vi "Init Search Page.vi"(7 "Next Button":refnum<vi>, 9 "\"Tab Backward To\" Refnum":refnum<vi>, 10 "\"Tab Forward To\" Refnum":refnum<vi>, 11 "SubPanel":refnum<vi>) -> (0 "Additional Search Ref":refnum<vi>, 1 "Next! Ref":refnum<vi>, 2 "Starter App Ref":refnum<vi>, 3 "Search Page Ref":refnum<vi>, 4 "SearchPage Ctrl #n Ref":refnum<vi>, 6 "SearchPage Ctrl #1 Ref":refnum<vi>)   [LabVIEW 2016]
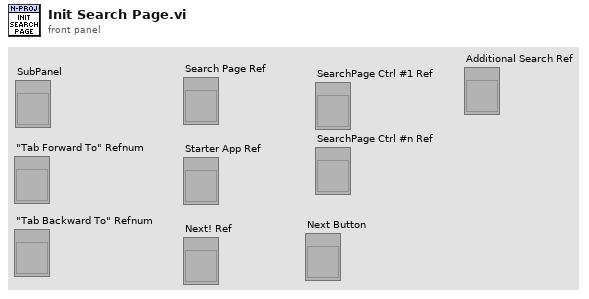
[diagram p1: front panel]
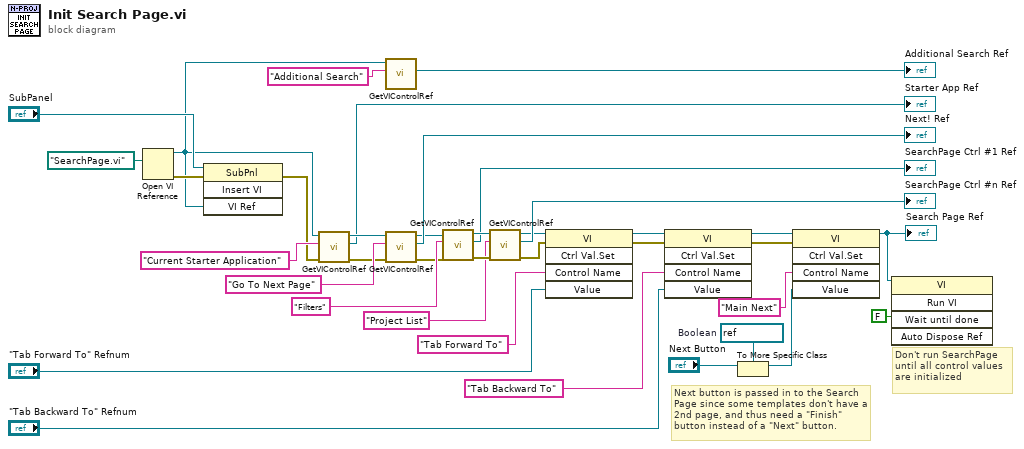
[diagram p0: block diagram]
diagram:
  w1 = refnum<vi> refnum  # Boolean
  # "Don't run SearchPage\nuntil all control values\nare initialized"
  # "Next button is passed in to the Search Page since some templates don't have a 2nd page, and thus need a \"Finish\" button instead of a \"Next\" button."
  n1 = Open VI Reference(vi path=path "SearchPage.vi") -> (vi reference=w7:refnum<vi>, error out=w29:errorcluster)  [unwired: 5 in]
  n2 = invoke on="Invoke Node" class="SubPnl" method="Insert VI"(reference="SubPanel", error in=w29, "VI Ref"=w7) -> (error out=w30:errorcluster)  [unwired: 1 in, 3 out]
  n3 = call <resource>:"GetVIControlRef.vi"("error in"=w30, "Control Name"="Current Starter Application", "VI Ref In"=w7) -> ("error out"=w33:errorcluster, "Control Reference"=→"Starter App Ref":refnum<vi>, "VI Ref Out"=w35:refnum<vi>)  [unwired: 6 in]
  n4 = call <resource>:"GetVIControlRef.vi"("Control Name"="Additional Search", "VI Ref In"=w7) -> ("Control Reference"=→"Additional Search Ref":refnum<vi>)  [unwired: 7 in, 2 out]
  n5 = call <resource>:"GetVIControlRef.vi"("error in"=w33, "Control Name"="Go To Next Page", "VI Ref In"=w35) -> ("error out"=w20:errorcluster, "Control Reference"=→"Next! Ref":refnum<vi>, "VI Ref Out"=w21:refnum<vi>)  [unwired: 6 in]
  n6 = call <resource>:"GetVIControlRef.vi"("error in"=w20, "Control Name"="Filters", "VI Ref In"=w21) -> ("error out"=w27:errorcluster, "Control Reference"=→"SearchPage Ctrl #1 Ref":refnum<vi>, "VI Ref Out"=w26:refnum<vi>)  [unwired: 6 in]
  n7 = call <resource>:"GetVIControlRef.vi"("error in"=w27, "Control Name"="Project List", "VI Ref In"=w26) -> ("error out"=w15:errorcluster, "Control Reference"=→"SearchPage Ctrl #n Ref":refnum<vi>, "VI Ref Out"=w17:refnum<vi>)  [unwired: 6 in]
  n8 = invoke class="VI" method="Ctrl Val.Set"(reference=w17, error in=w15, "Control Name"="Tab Forward To" ("name or relative path"), "Value"="\"Tab Forward To\" Refnum") -> (reference out=w14:refnum<vi>, error out=w13:errorcluster)  [unwired: 1 in, 3 out]
  n9 = invoke class="VI" method="Ctrl Val.Set"(reference=w14, error in=w13, "Control Name"="Tab Backward To", "Value"="\"Tab Backward To\" Refnum") -> (reference out=w11:refnum<vi>, error out=w10:errorcluster)  [unwired: 1 in, 3 out]
  n10 = To More Specific Class(target class=w1, reference="Next Button") -> (specific class reference=w2:refnum<vi>)  [unwired: 1 in, 1 out]
  n11 = invoke class="VI" method="Ctrl Val.Set"(reference=w11, error in=w10, "Control Name"="Main Next", "Value"=w2) -> (reference out=w3:refnum<vi>)  [unwired: 1 in, 4 out]
  "Search Page Ref" <- w3
  n12 = invoke class="VI" method="Run VI"(reference=w3, "Wait until done"=FALSE ("Wait Until Done")) -> ()  [unwired: 3 in, 5 out]
